vi "createCommand.vi"(8 "error in (no error)":errorcluster, 9 "CommandValue":T1, 10 "CommandID":i32) -> (0 "error out":errorcluster, 3 "InternalCommandId out":refnum<class "InternalCommandId.lvclass">)   [LabVIEW 2016, in "InternalCommandId.lvclass"]
uses:
  InternalCommandId.lvclass
  ts_electrometeruserevents/Typedefs/CommandValue.ctl
  InternalCommandId.lvclass/InternalCommandId.ctl
  ts_electrometeruserevents/Typedefs/ElectrometerTypedefs.lvlib
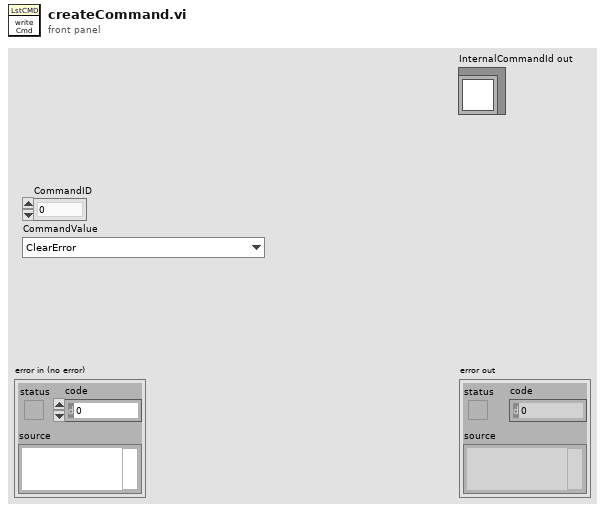
[diagram p1: front panel]
types:
  T1 = typedef "ElectrometerTypedefs.lvlib/CommandValue.ctl" = enum16{"ClearError", "Disable", "Enable", "Exit", "GoToStandby", "OnHeartbeat", "OnIncomingMessagingError", "OnInterrupt", "Start", "SetDigitalFilter", "StartScan", "StartScanDt", "StartScanReachIntensity", "StopScan", "SetIntegrationTime", "PerformZeroCalib", "SetRange", "SetMode", "Power"}
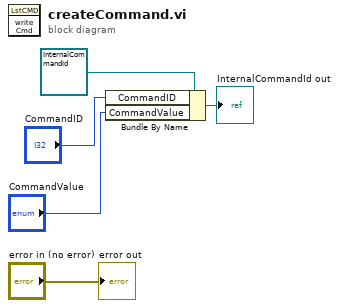
[diagram p0: block diagram]
diagram:
  n1 = Bundle By Name(cluster=refnum<class "InternalCommandId.lvclass"> refnum ("InternalCommandId in"), "CommandID"="CommandID", "CommandValue"="CommandValue") -> (→"InternalCommandId out":refnum<class "InternalCommandId.lvclass">)
  "error out" <- "error in (no error)"
